vi "Inclinometer Graph View.vi"(8 "M1M3 Support Events in":refnum<class "M1M3 Support Events.lvclass">) -> ()   [LabVIEW 2016, in "M1M3SupportEUI_Views.lvlib"]
uses:
  M1M3SupportEUI_Views.lvlib
  M1M3 Support Events/M1M3 Support Events.lvclass
  M1M3 Support Events/M1M3 Support Events.lvclass/M1M3 Support Events.ctl
  Typedefs/StateTypes.ctl
  Typedefs/M1M3SupportEUI_TypeDefs.lvlib
panel:
  out "XY Graph":cluster{dbl[], dbl[]}(graph)
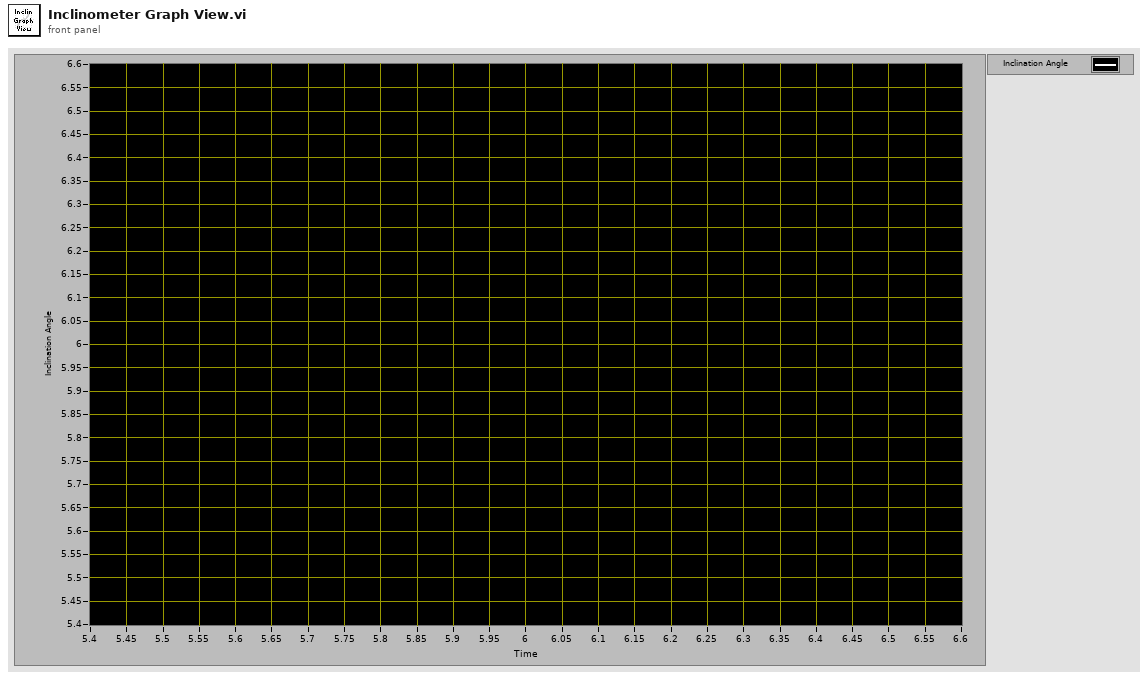
[diagram p1: front panel]
types:
  T1 = typedef "M1M3SupportEUI_TypeDefs.lvlib/M1M3 Support Events.ctl" = cluster{"M1M3 Support State":refnum<user-event>, "Inclinometer  Data":refnum<user-event>, "IMS Data":refnum<user-event>}
  T2 = typedef "M1M3SupportEUI_TypeDefs.lvlib/StateTypes.ctl" = enum16{"Offline State", "Fault State", "Standby State", "Disabled State", "Enabled State", "Wait For User Input State", "Test Actuator State"}
  T3 = cluster{"Timestamp Out":dbl[], "Inclination Angle Out":dbl[]}
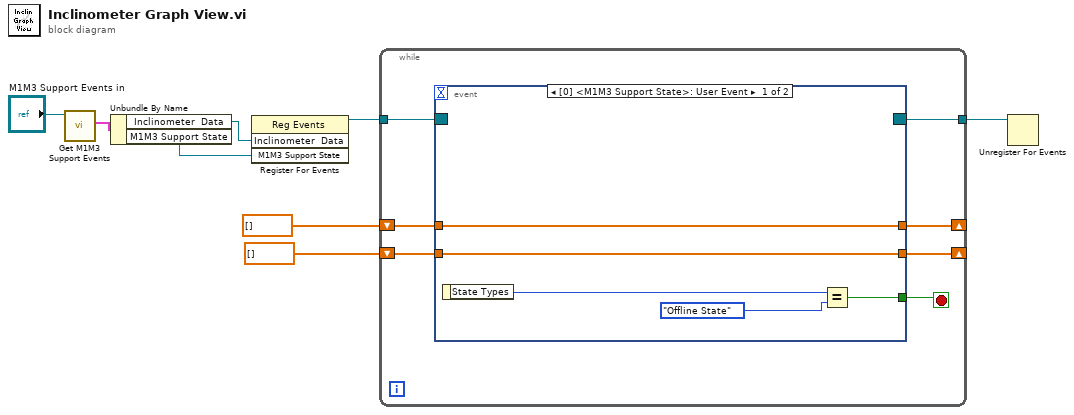
[diagram p0: block diagram]
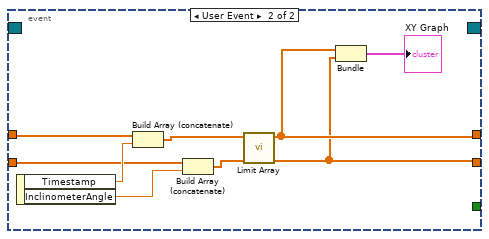
[diagram p2: hidden frame]
diagram:
  n1 = call "Get M1M3 Support Events.vi"("M1M3 Support Events in"="M1M3 Support Events in") -> ("M1M3 Support Events"=w7:T1)  [unwired: 9 in, 1 out]
  n2 = Unbundle By Name(w7) -> ("Inclinometer  Data"=w6:refnum<user-event>, "M1M3 Support State"=w1:refnum<user-event>)
  n3 = register-events(w6, w1) -> (reference out=w5:refnum<event-registration>)  [unwired: 2 in, 1 out]
  n4 = while {
    tunnel: w5 -> [w15]
    tunnel: [w14] -> w4
    shift-right: [w11] -> _
    shift-left: dbl[] [] -> [w12]
    shift-right: [w9] -> _
    shift-left: dbl[] [] -> [w10]
    stop <- w13 stop-if-true
    n5 = event shown="[0] <M1M3 Support State>: User Event" {
      selector: w15 -> [_ _]
      dyn-events: [_ _] -> w14
      timeout: _ -> [_ _]
      tunnel: [w18 _] -> w13
      tunnel: w12 -> [w16 w29]
      tunnel: [w16 w23] -> w11
      tunnel: w10 -> [w17 w27]
      tunnel: [w17 w21] -> w9
      event User Event {
        n6 = event-data() -> ("State Types"=w20:T2)  [unwired: 1 in]
        n7 = Equal?(x=w20, y=StateTypes."Offline State" ("State Types")) -> (x = y?=w18:bool)
      }
      event User Event {
        n8 = event-data() -> ("Timestamp"=w28:dbl, "InclinometerAngle"=w26:dbl)  [unwired: 1 in]
        n9 = Build Array (concatenate)(w29, w28) -> (w24:dbl[])
        n10 = Build Array (concatenate)(w27, w26) -> (w22:dbl[])
        n11 = call "Limit Array.vi"("Inclination Angle In"=w22, "Timestamp In"=w24) -> ("Inclination Angle Out"=w21:dbl[], "Timestamp Out"=w23:dbl[])  [unwired: 8 in]
        n12 = Bundle("Timestamp Out"=w23, "Inclination Angle Out"=w21) -> (→"XY Graph":T3)  [unwired: 1 in]
      }
    }
  }
  n13 = Unregister For Events(event registration refnum=w4) -> ()  [unwired: 1 in, 1 out]
